vi "SR830 query reference mode.vi"(8 "error in (no error)":errorcluster, 11 "VISA resource name":refnum<visa-resource-name>) -> (0 "error out":errorcluster, 2 "reference mode":enum16{"external", "internal"}(ring), 3 "VISA resource name out":refnum<visa-resource-name>)   [LabVIEW 2017, in "SR830.lvlib"]
doc: "Reads the current reference mode (internal or external) of the lock-in amplifier."
uses:
  SR830.lvlib
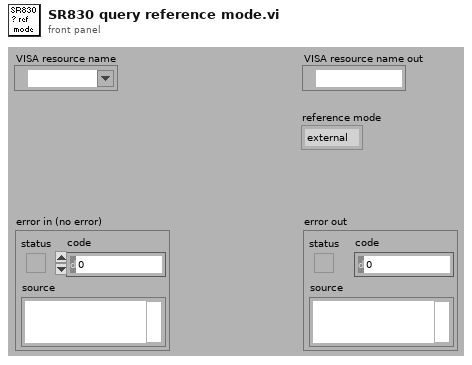
[diagram p1: front panel]
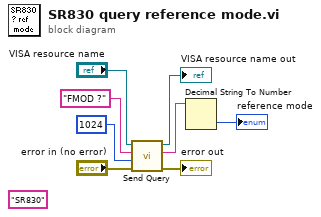
[diagram p0: block diagram]
diagram:
  (unwired) "SR830" ("name (unnamed)")
  n1 = call "Send Query.vi"("error in (no error)"="error in (no error)", "Bytes Count"=u32 1024 ("bytes to read (1000)"), "write buffer"="FMOD ?", "VISA resource name"="VISA resource name") -> ("error out"=→"error out":errorcluster, "read buffer"=w3:string, "VISA resource name out"=→"VISA resource name out":refnum<visa-resource-name>)  [unwired: 5 in]
  n2 = Decimal String To Number(string=w3) -> (number=→"reference mode":i32)  [unwired: 3 out]
